vi "General-InsertContrastInFile.vi"(2 "error IN":errorcluster, 3 "contraste":dbl, 4 "tiempo (ms)":u32, 5 "refnum IN":refnum<file>) -> (0 "error OUT":errorcluster, 1 "refnum OUT":refnum<file>)   [LabVIEW 2010]
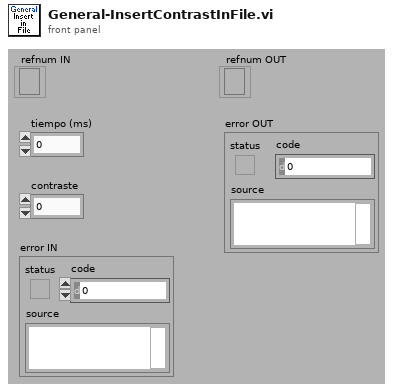
[diagram p1: front panel]
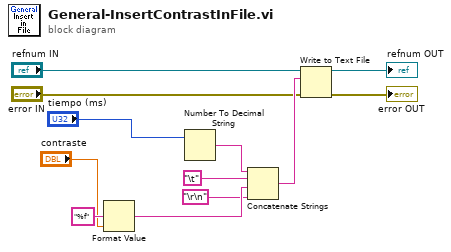
[diagram p0: block diagram]
diagram:
  n1 = Format Value(format string="%f", value (0)="contraste") -> (output string=w11:string)  [unwired: 1 in]
  n2 = Number To Decimal String(number="tiempo (ms)") -> (decimal integer string=w7:string)  [unwired: 1 in]
  n3 = Concatenate Strings(w7, "\t", w11, "\r\n") -> (w9:string)
  n4 = Write to Text File(file (use dialog)="refnum IN", text=w9, error in="error IN") -> (refnum out=→"refnum OUT":refnum<file>, error out=→"error OUT":errorcluster)  [unwired: 1 in, 1 out]
